vi "Set Osc Sample.vi"(11 "sample":u32) -> (3 "function return":u32)   [LabVIEW 2021, in "vmmso.lvlib"]
doc: "DLL_API unsigned int WINAPI SetOscSample(unsigned int sample);"
uses:
  vmmso.lvlib
  vmmso.dll
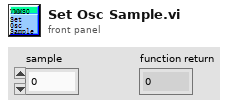
[diagram p1: front panel]
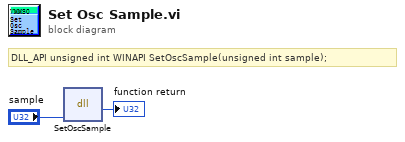
[diagram p0: block diagram]
diagram:
  # "DLL_API unsigned int WINAPI SetOscSample(unsigned int sample);"
  n1 = dll-call lib="D:/labviewdemo/LabviewDemo 21/vmmso/vmmso.*" fn="SetOscSample"("sample"="sample") -> (→"function return":u32)  [unwired: 4 in, 2 out]
